vi "getLabel.vi"(8 "error in (no error)":errorcluster, 11 "Delay in":refnum<class "Delay.lvclass">) -> (0 "error out":errorcluster, 2 "label":string, 3 "Delay out":refnum<class "Delay.lvclass">)   [LabVIEW 2011, in "Tools.lvlib" / "Scripting.lvlib" / "Delay.lvclass"]
uses:
  Delay.lvclass
  Delay.lvclass/Delay.ctl
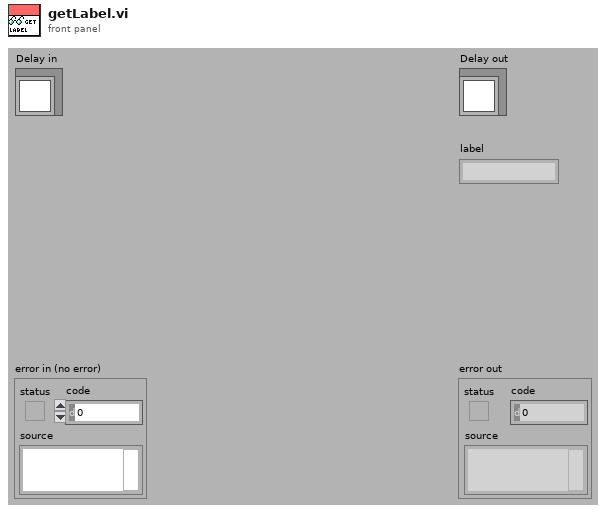
[diagram p1: front panel]
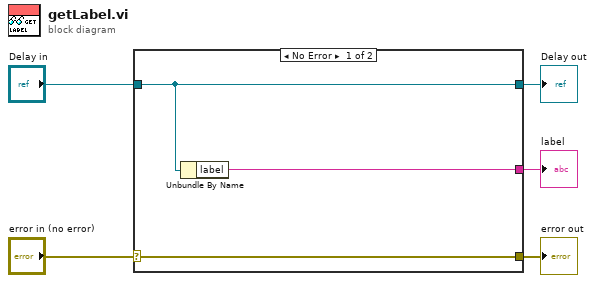
[diagram p0: block diagram]
diagram:
  n1 = case shown="No Error" "error in (no error)" {
    selector: "error in (no error)" -> [w8 w9]
    tunnel: [w8 w9] -> w4
    tunnel: [w7 w10] -> w2
    tunnel: "Delay in" -> [w7 w10]
    tunnel: [w6 _] -> w1
    frame No Error {
      n2 = Unbundle By Name(w7) -> ("label"=w6:string)
    }
    frame Error {
    }
  }
  "error out" <- w4
  "Delay out" <- w2
  "label" <- w1
